vi "Write Timing Source dt.vi"(8 "error in":errorcluster, 10 "Timing Source dt":u32, 11 "Standard Engine Repo Data in":refnum<class "synchronous engine configuration.lvclass">) -> (0 "error out":errorcluster, 3 "Standard Engine Repo Data out":refnum<class "synchronous engine configuration.lvclass">)   [LabVIEW 2013, in "synchronous engine configuration.lvclass"]
uses:
  synchronous engine configuration.lvclass
  synchronous engine configuration.lvclass/synchronous engine configuration.ctl
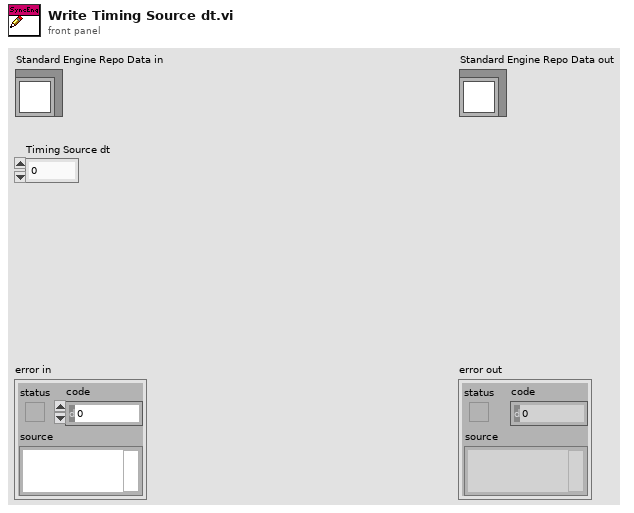
[diagram p1: front panel]
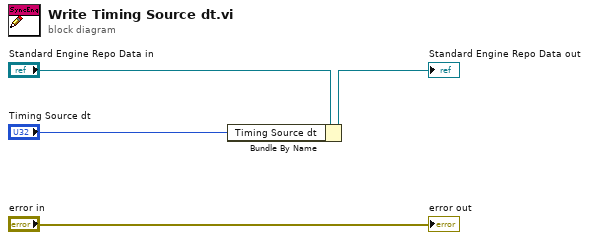
[diagram p0: block diagram]
diagram:
  n1 = Bundle By Name(cluster="Standard Engine Repo Data in", "Timing Source dt"="Timing Source dt") -> (→"Standard Engine Repo Data out":refnum<class "synchronous engine configuration.lvclass">)
  "error out" <- "error in"
